vi "TeamMove (Private).vi"(8 "error in (no error)":errorcluster, 11 "TeamEffort in":refnum<class "TeamEffort.lvclass">) -> (0 "error out":errorcluster, 3 "TeamEffort out":refnum<class "TeamEffort.lvclass">)   [LabVIEW 2015, in "TeamEffort.lvclass"]
uses:
  TeamEffort.lvclass
  TeamEffort.lvclass/TeamEffort.ctl
  Player Cluster.ctl
  Team Move Input.ctl
  Type Defs/Action Enum.ctl
  Team Move Output.ctl
  Type Defs/Direction Enum.ctl
  Square/Square.lvclass
  Type Defs/SB Type Defs.lvlib
panel:
  out "Intensity Graph":i32[][](graph)
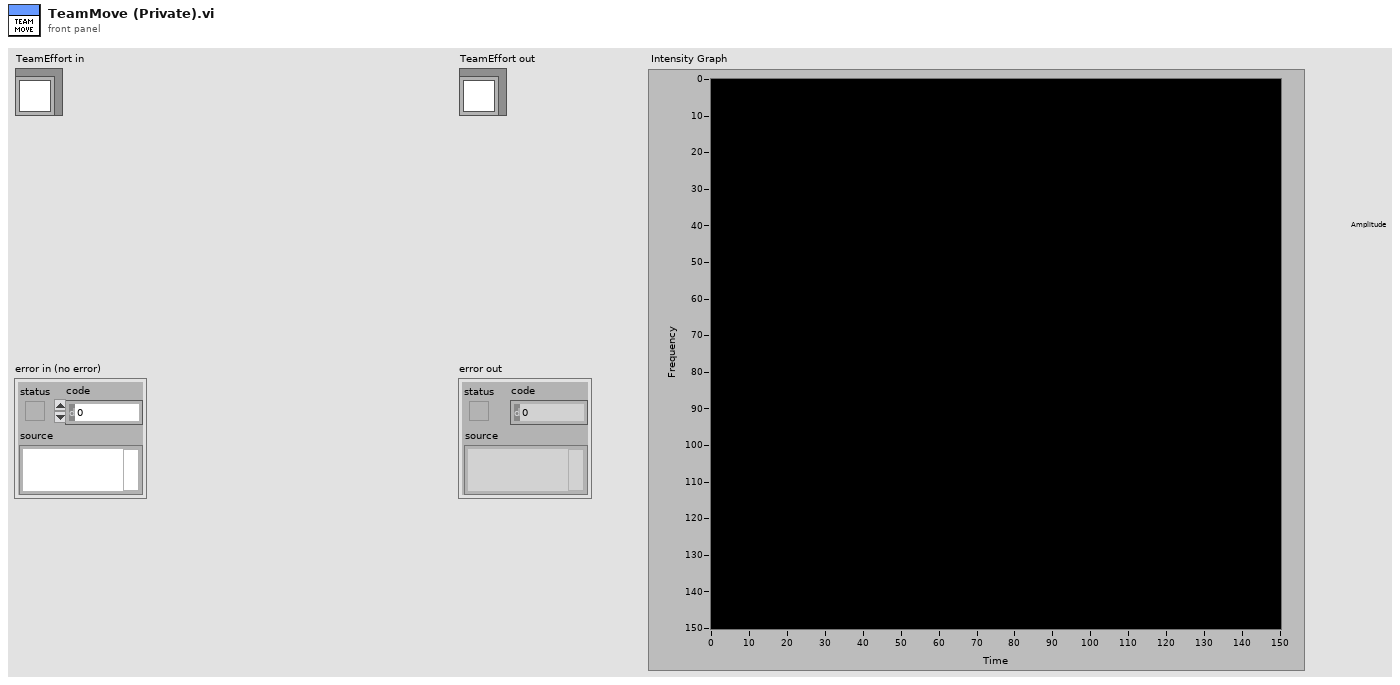
[diagram p1: front panel]
types:
  T1 = typedef "TeamEffort.lvclass/Player Cluster.ctl" = cluster{"Exp. Move":i32, "Moved?":bool, "In":T2, "Out":T4}
  T2 = typedef "TeamEffort.lvclass/Team Move Input.ctl" = cluster{"PlayerID":i32, "Y":i32, "X":i32, "Last Move":i32, "LastAction":T3}
  T3 = typedef "SB Type Defs.lvlib/Action Enum.ctl" = enum16{"Wait", "Move", "Attack", "Replicate"}
  T4 = typedef "TeamEffort.lvclass/Team Move Output.ctl" = cluster{"Action":T3, "Direction":T5, "Replicated":refnum<class "Square.lvclass">}
  T5 = typedef "SB Type Defs.lvlib/Direction Enum.ctl" = enum16{"NW", "N", "NE", "E", "SE", "S", "SW", "W"}
  T6 = typedef "TeamEffort.lvclass/Grid Cluster.ctl" = cluster{"p[x][y]":i32[][], "Move Count":i32, "Info[p]":T1[], "Known_p":i32}
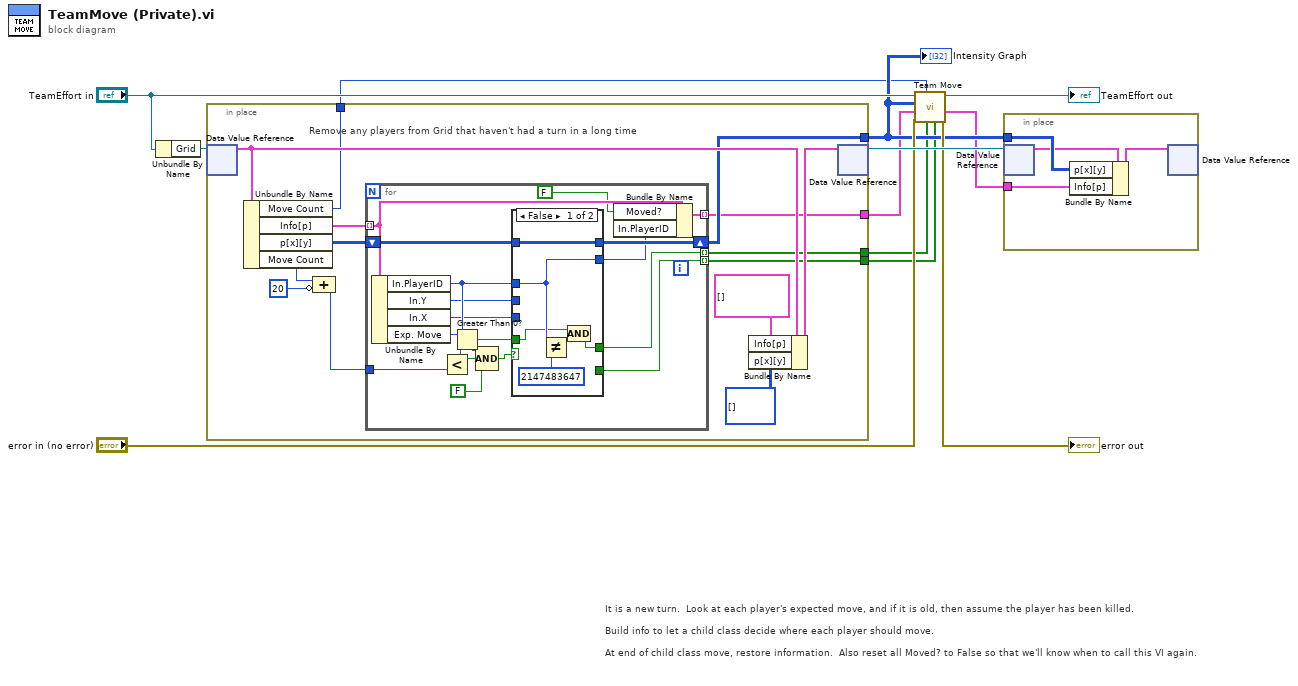
[diagram p0: block diagram]
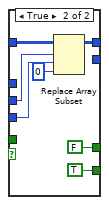
[diagram p2: hidden frame]
diagram:
  # "It is a new turn.  Look at each player's expected move, and if it is old, then assume the player has been killed.\n\nBuild info to let a child class decide where each player should move.\n\nAt end of child class move, restore information.  Also reset all Moved? to False so that we'll know when to call this VI again."
  n1 = Unbundle By Name("TeamEffort in") -> ("Grid"=w12:refnum<data-value>)
  n2 = in-place {
    in-place-border: [w21] -> w6
    in-place-border: [w17] -> w5
    in-place-border: [w15] -> w2
    in-place-border: [w14] -> w4
    in-place-border: [w13] -> w3
    # "Remove any players from Grid that haven't had a turn in a long time"
    n3 = in-place-dvr #1(w12) -> (w26:T6)  [unwired: 1 out]
    n4 = Unbundle By Name(w26) -> ("Move Count"=w17:i32, "Info[p]"=w19:T1[], "p[x][y]"=w18:i32[][], "Move Count"=w24:i32)
    n5 = Compound Arithmetic op=ADD(w24, invert 20 ("value")) -> (w22:i32)
    n6 = for {
      tunnel: w19 -> [w29] mode=indexing
      tunnel: w22 -> [w43]
      shift-right: [w38] -> w21
      shift-left: w18 -> [w41]
      tunnel: [w36] -> w15 mode=indexing
      tunnel: [w31] -> w14 mode=indexing
      tunnel: [w30] -> w13 mode=indexing
      n7 = Unbundle By Name(w29) -> ("In.PlayerID"=w39:i32, "In.Y"=w33:i32, "In.X"=w32:i32, "Exp. Move"=w28:i32)
      n8 = Less?(x=w28, y=w43) -> (x < y?=w42:bool)
      n9 = Greater Than 0?(x=w39) -> (x > 0?=w37:bool)
      n10 = Compound Arithmetic op=AND(w37, w42, FALSE ("value")) -> (w40:bool)
      n11 = case shown="False" w40 {
        tunnel: w41 -> [w49 w56]
        tunnel: w39 -> [w48 _]
        tunnel: w33 -> [_ w53]
        tunnel: w32 -> [_ w52]
        tunnel: [_ TRUE] -> w30
        tunnel: [w44 FALSE] -> w31
        tunnel: [w49 w50] -> w38
        tunnel: w37 -> [w46 _]
        tunnel: [w48 _] -> w35
        frame False {
          n12 = Not Equal?(x=w48, y=2147483647 ("value")) -> (x != y?=w45:bool)
          n13 = Compound Arithmetic op=AND(w46, w45) -> (w44:bool)
        }
        frame True {
          n14 = Replace Array Subset(array=w56, new element=0 ("new element/subarray"), index (row)=w53, index (col)=w52) -> (w50:i32[][])
        }
      }
      n15 = Bundle By Name(cluster=w29, "Moved?"=FALSE, "In.PlayerID"=w35) -> (w36:T1)
    }
    n16 = Bundle By Name(cluster=w26, "Info[p]"=T1[] [], "p[x][y]"=i32[][] []) -> (w25:T6)
    n17 = in-place-dvr #1(w25) -> (w10:refnum<data-value>)  [unwired: 1 out]
  }
  "Intensity Graph" <- w6
  n18 = call-dynamic "Team Move.vi"("MIA?[p]"=w3, "Confirmed?[p]"=w4, "Move Cnt"=w5, "error in (no error)"="error in (no error)", "Player[p] in"=w2, "p[x][y]"=w6, "TeamEffort in"="TeamEffort in") -> ("error out"=→"error out":errorcluster, "Player[p] out"=w1:T1[], "TeamEffort out"=→"TeamEffort out":refnum<class "TeamEffort.lvclass">)  [unwired: 2 in]
  n19 = in-place {
    in-place-border: w6 -> [w60]
    in-place-border: w1 -> [w57]
    n20 = in-place-dvr #2(w10) -> (w58:T6)  [unwired: 1 out]
    n21 = Bundle By Name(cluster=w58, "p[x][y]"=w60, "Info[p]"=w57) -> (w59:T6)
    n22 = in-place-dvr #2(w59) -> ()  [unwired: 2 out]
  }
